vi "example-SequentialFileName.vi"() -> ()   [LabVIEW 2021]
panel:
  in  "String to Save":string
  in  "File Name":path
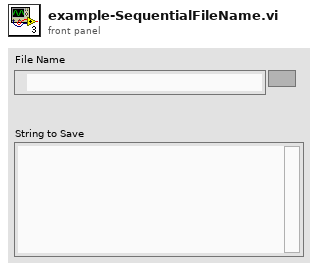
[diagram p1: front panel]
types:
  T1 = enum16{"open", "replace", "create", "open or create", "replace or create", "replace or create with confirmation"}
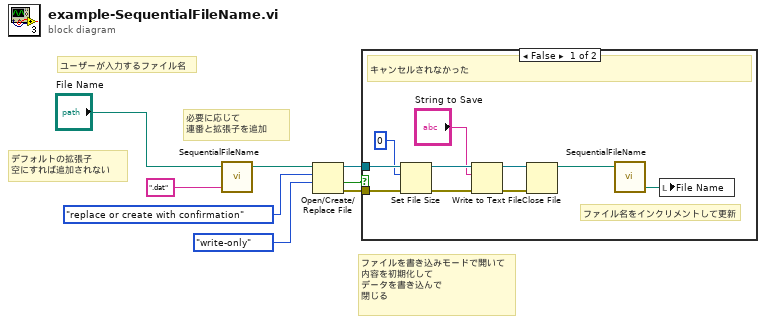
[diagram p0: block diagram]
diagram:
  # "ファイルを書き込みモードで開いて\n内容を初期化して\nデータを書き込んで\n閉じる"
  # "ユーザーが入力するファイル名"
  # "デフォルトの拡張子\n空にすれば追加されない"
  # "必要に応じて\n連番と拡張子を追加"
  n1 = call "SequentialFileName.vi"("Extention (.dat)"=".dat", "File Name In"="File Name") -> ("File Name With Sequence"=w3:path)  [unwired: 2 in, 1 out]
  n2 = Open/Create/Replace File(file path (use dialog)=w3, operation (0:open)=T1."replace or create with confirmation" ("操作 (0:open)"), access (0:read/write)=enum16{"read/write", "read-only", "write-only"}."write-only" ("アクセス (0:read/write)")) -> (refnum out=w8:refnum<file>, cancelled=w1:bool, error out=w5:errorcluster)  [unwired: 3 in]
  n3 = case shown="False" w1 {
    tunnel: w8 -> [w18 _]
    tunnel: w5 -> [w17 _]
    frame False {
      # "ファイル名をインクリメントして更新"
      # "キャンセルされなかった"
      n4 = Set File Size(4:w17, 6:i64 0 ("サイズ (バイト)"), 7:w18) -> (0:w11:errorcluster, 3:w16:refnum<file>)
      n5 = Write to Text File(file (use dialog)=w16, text="String to Save", error in=w11) -> (refnum out=w14:refnum<file>, error out=w13:errorcluster)  [unwired: 1 in, 1 out]
      n6 = Close File(refnum=w14, error in=w13) -> (path=w10:path)  [unwired: 1 out]
      n7 = call "SequentialFileName.vi"("File Name In"=w10) -> ("Next File Name"=w9:path)  [unwired: 3 in, 1 out]
      n8 = local write "File Name"(w9) -> ()
    }
    frame True {
    }
  }
